vi "Greyscale Data to ARGB Data.vi"(1 "Greyscale Data":u8[][](array[numeric])) -> (0 "ARGB Data":u32[][](array[numeric]) format="%.0x")   [LabVIEW 2020, in "image.lvlib"]
doc: "Convert Greyscale Data to ARGB Data."
uses:
  image.lvlib
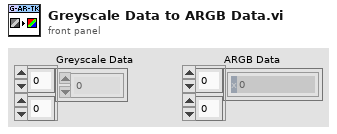
[diagram p1: front panel]
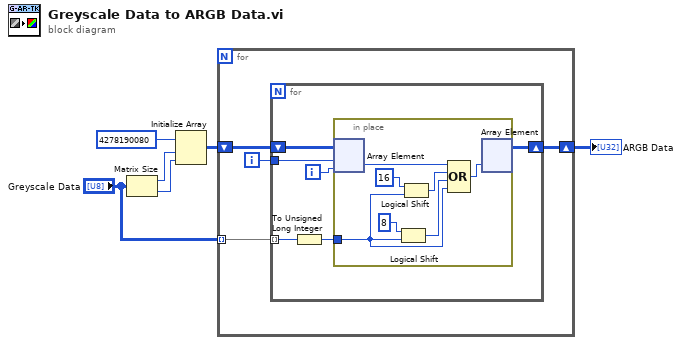
[diagram p0: block diagram]
diagram:
  n1 = Matrix Size(0:"Greyscale Data") -> (1:w6:i32, 2:w5:i32)
  n2 = Initialize Array(u32 4278190080, w6, w5) -> (w3:u32[][])
  n3 = for {
    shift-right: [w8] -> w2
    shift-left: w3 -> [w10]
    tunnel: "Greyscale Data" -> [w7] mode=indexing
    i -> [w9]
    n4 = for {
      shift-right: [w13] -> w8
      shift-left: w10 -> [w16]
      tunnel: w9 -> [w15]
      tunnel: w7 -> [w12] mode=indexing
      i -> [w14]
      n5 = To Unsigned Long Integer(number=w12) -> (unsigned 32bit integer=w11:u32)
      n6 = in-place {
        in-place-border: w11 -> [w19]
        n7 = in-place-array #1(w16, w15, w14) -> (w23:u32)
        n8 = Logical Shift(y=i16 8, x=w19) -> (x << y=w22:u32)
        n9 = Logical Shift(y=i16 16, x=w19) -> (x << y=w20:u32)
        n10 = Compound Arithmetic op=OR(w23, w20, w22, w19) -> (w17:u32)
        n11 = in-place-array #1(w17) -> (w13:u32[][])  [unwired: 2 out]
      }
    }
  }
  "ARGB Data" <- w2
